vi "GlobalSetGetPositionParameters.vi"() -> ()   [LabVIEW 2013]
panel:
  out "ind POS X rad 2":dbl
  out "ind POS  Y rad 2":dbl
  out "ind POS Z 2":dbl
  out "ind POS X 2":dbl
  out "ind POS  Y 2":dbl
  in  "POS X rad":dbl
  in  "POS  Y rad":dbl
  out "ScanTime":dbl
  in  "POS Z":dbl
  in  "POS X":dbl
  in  "POS  Y":dbl
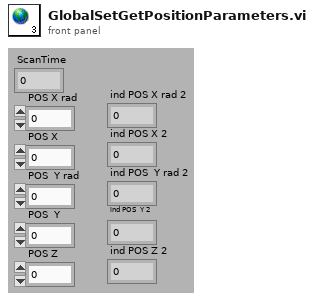
[diagram p1: front panel]
diagram:
